vi "GVStringArray.vi"() -> ()   [LabVIEW 2010]
panel:
  in  "String":string
  in  "Array":string[](array[string])
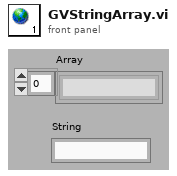
[diagram p1: front panel]
diagram:
